vi "CuatroLinea.vi"() -> ()   [LabVIEW 2020]
uses:
  Downloads/TTT2011/Symbol.ctl
  Control 13.ctl
panel:
  out "Whos Turn?":string
  in  "Array":T1[][](array[typedef])
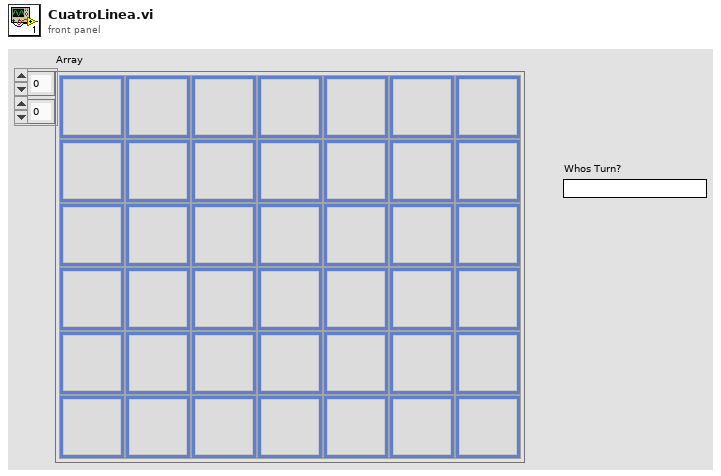
[diagram p1: front panel]
types:
  T1 = typedef "Control 13.ctl" = u16
  T2 = typedef "Symbol.ctl" = u16
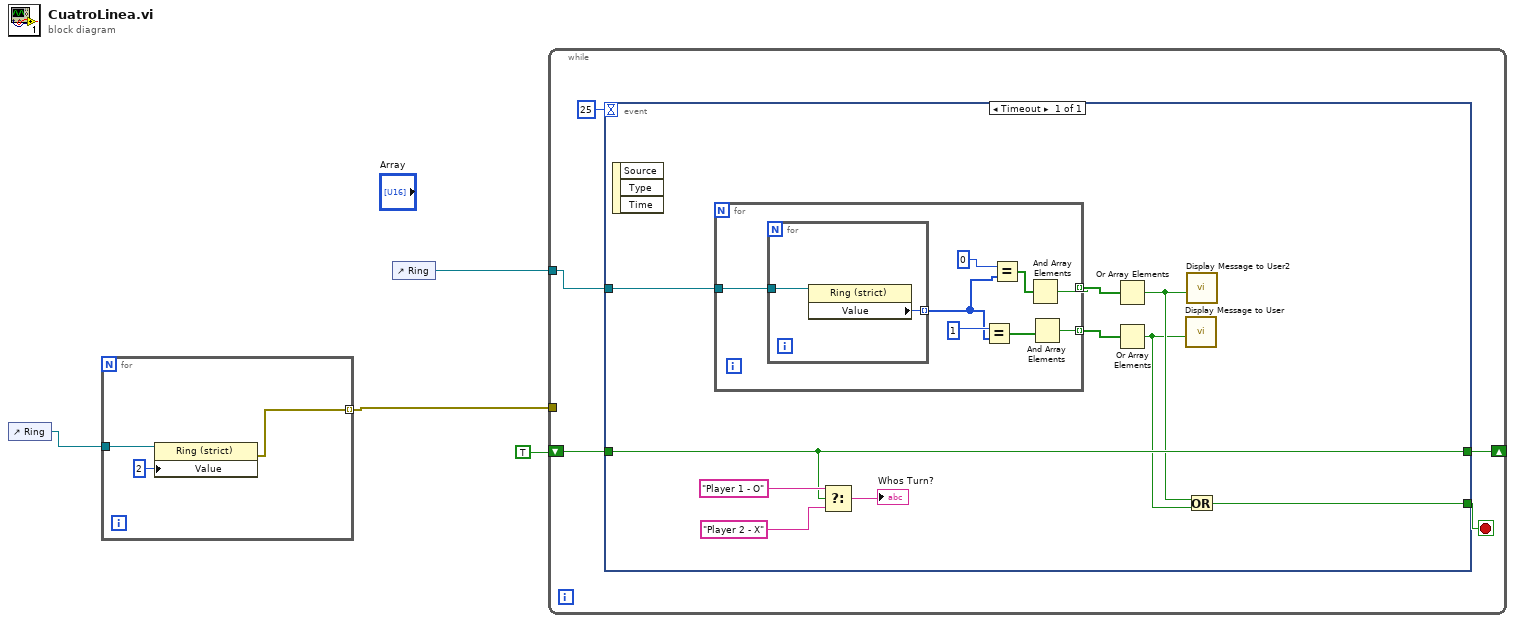
[diagram p0: block diagram]
diagram:
  n1 = control-ref of="Ring"() -> (w3:refnum<vi>)
  n2 = for {
    tunnel: w3 -> [w7]
    tunnel: [w5] -> w2 mode=indexing
    n3 = property class="Ring (strict)"(reference=w7, "Value"=T1 2) -> (error out=w5:errorcluster)  [unwired: 1 in, 1 out]
  }
  n4 = control-ref of="Ring"() -> (w1:refnum<vi>)
  n5 = while {
    shift-right: [w11] -> _
    shift-left: TRUE -> [w12]
    tunnel: w2 -> [_]
    tunnel: w1 -> [w8]
    stop <- w10 stop-if-true
    n6 = event shown="[0] Timeout" {
      selector: _ -> [_]
      dyn-events: _ -> [_]
      timeout: 25 -> [_]
      tunnel: w12 -> [w17]
      tunnel: [w17] -> w11
      tunnel: [w14] -> w10
      tunnel: w8 -> [w13]
      event Timeout {
        n7 = event-data() -> ()  [unwired: 1 in, 3 out]
        n8 = for {
          tunnel: [w26] -> w22 mode=indexing
          tunnel: [w24] -> w21 mode=indexing
          tunnel: w13 -> [w23]
          n9 = for {
            tunnel: [w32] -> w28 mode=indexing
            tunnel: w23 -> [w31]
            n10 = property class="Ring (strict)"(reference=w31) -> ("Value"=w32:T1)  [unwired: 1 in, 2 out]
          }
          n11 = Equal?(x=T2 1 ("Value"), y=w28) -> (x = y?=w25:bool[])
          n12 = Equal?(x=T2 0 ("Value"), y=w28) -> (x = y?=w27:bool[])
          n13 = And Array Elements(Boolean array=w27) -> (logical AND=w26:bool)
          n14 = And Array Elements(Boolean array=w25) -> (logical AND=w24:bool)
        }
        n15 = Select(t="Player 1 - O", s=w17, f="Player 2 - X") -> (s? t:f=→"Whos Turn?":string)
        n16 = Or Array Elements(Boolean array=w22) -> (logical OR=w16:bool)
        n17 = Or Array Elements(Boolean array=w21) -> (logical OR=w15:bool)
        n18 = call "Display Message to User"("Enable"=w15) -> ()  [unwired: 9 in, 2 out]
        n19 = call "Display Message to User2"("Enable"=w16) -> ()  [unwired: 9 in, 2 out]
        n20 = Or(x=w16, y=w15) -> (x .or. y?=w14:bool)
      }
    }
  }
